vi "read_pressures.vi"(10 "press task in":refnum<k21>, 11 "Channel 1":tag) -> (2 "press task out":refnum<k21>, 3 "Ch. 1 value":dbl format="%0.2f")   [LabVIEW 2014]
uses:
  <vilib>/DAQmx/create/channels.llb/DAQmx Create Channel (AI-Voltage-Basic).vi
  <vilib>/DAQmx/configure/trigger.llb/DAQmx Start Trigger (None).vi
  <vilib>/DAQmx/read.llb/DAQmx Read (Analog 1D DBL NChan 1Samp).vi
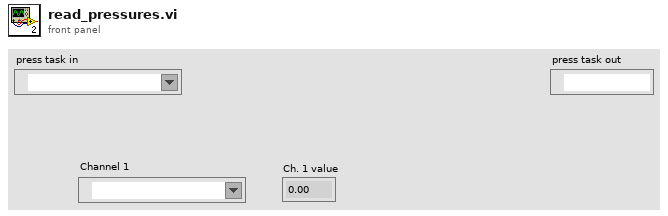
[diagram p1: front panel]
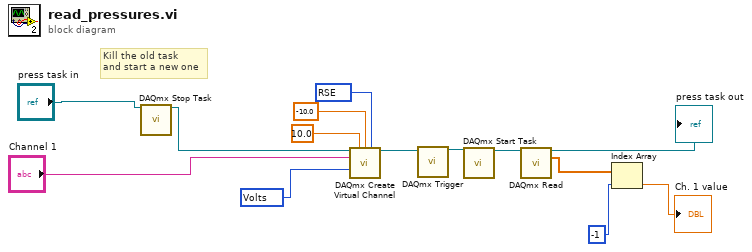
[diagram p0: block diagram]
diagram:
  w9 = 10083 items=["default"=-1, "RSE"=10083, "NRSE"=10078, "Differential"=10106, "Pseudodifferential"=12529] ("input terminal configuration")
  w11 = 10348 items=["Volts"=10348, "From Custom Scale"=10065] ("units")
  # "Kill the old task\nand start a new one"
  n1 = call <vilib>:"DAQmx Stop Task.vi"("task/channels in"="press task in") -> ("task out"=w3:refnum<k21>)  [unwired: 13 in, 1 out]
  n2 = call-poly <vilib>:"DAQmx Create Virtual Channel.vi"("task in"=w3, "maximum value"=10.0, "minimum value"=-10.0, "input terminal configuration"=w9, "physical channels"="Channel 1", "units"=w11) -> ("task out"=w2:refnum<k21>)  [unwired: 8 in, 1 out]
  n3 = call-poly <vilib>:"DAQmx Trigger.vi"("task/channels in"=w2) -> ("task out"=w1:refnum<k21>)  [unwired: 13 in, 1 out]
  n4 = call <vilib>:"DAQmx Start Task.vi"("task/channels in"=w1) -> ("task out"=w10:refnum<k21>)  [unwired: 13 in, 1 out]
  n5 = call-poly <vilib>:"DAQmx Read.vi"("task/channels in"=w10) -> ("task out"=→"press task out":refnum<k21>, "data"=w6:dbl[])  [unwired: 12 in, 1 out]
  n6 = Index Array(array=w6, index=-1) -> (element=→"Ch. 1 value":dbl)
